vi "Create Object.vi"   [LabVIEW 2017, in "NI_3D Picture Control.lvlib"]
doc: "Creates a new 3D object to display in the 3D scene."
uses:
  <vilib>/picture/3D Picture Control/NI_3D Picture Control.lvlib
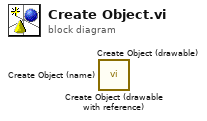
[diagram p0: block diagram]
diagram:
  n1 = call <vilib>:"Create Object (drawable with reference).vi"() -> ()  [unwired: 9 in, 3 out]
  n2 = call <vilib>:"Create Object (drawable).vi"() -> ()  [unwired: 10 in, 2 out]
  n3 = call <vilib>:"Create Object (name).vi"() -> ()  [unwired: 10 in, 2 out]
